vi "SI100_R1.vi"() -> ()   [LabVIEW 2022 SP3, in "SI100_ReactorTemperatureRise.lvclass"]
uses:
  SI100_ReactorTemperatureRise.lvclass
  SI100_ReactorTemperatureRise.lvclass/SI100_ReactorTemperatureRise.ctl
  SIClass/SIClass.lvclass
panel:
  out "SIClass out 4":refnum<class "SIClass.lvclass">
  out "SIClass out 3":refnum<class "SIClass.lvclass">
  out "SIClass out 2":refnum<class "SIClass.lvclass">
  out "SIClass out":refnum<class "SIClass.lvclass">
  in  "error in":errorcluster
  out "T-Rise 2nd Max":dbl
  in  "3 JEC20 CT951 XQ01":dbl
  in  "Loop ID 4":enum16{"10", "20", "30", "40"}(ring)
  in  "3 JEC20 CT954 XQ01":dbl
  in  "Loop ID 3":enum16{"10", "20", "30", "40"}(ring)
  in  "3 JEC20 CT953 XQ01":dbl
  in  "Loop ID 2":enum16{"10", "20", "30", "40"}(ring)
  in  "3 JEC10 CT952 XQ01":dbl
  in  "Loop ID":enum16{"10", "20", "30", "40"}(ring)
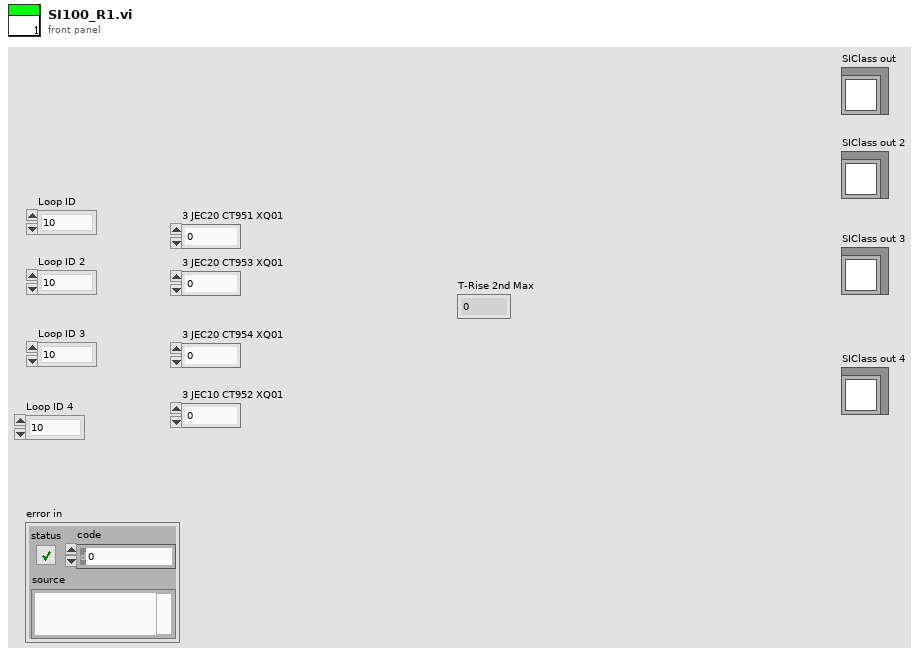
[diagram p1: front panel]
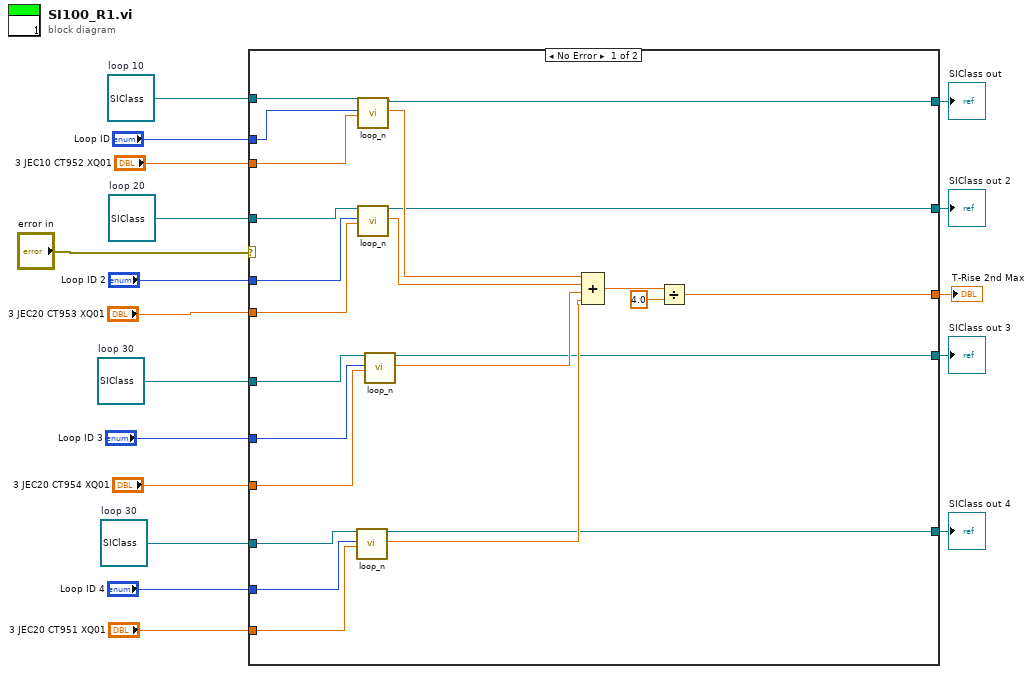
[diagram p0: block diagram]
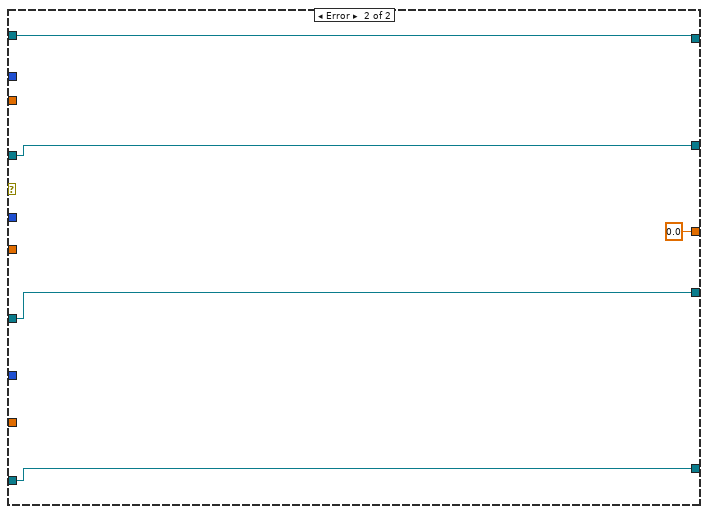
[diagram p2: hidden frame]
diagram:
  w7 = refnum<class "SIClass.lvclass"> refnum  # loop 30
  w10 = refnum<class "SIClass.lvclass"> refnum  # loop 30
  w15 = refnum<class "SIClass.lvclass"> refnum  # loop 20
  w18 = refnum<class "SIClass.lvclass"> refnum  # loop 10
  n1 = case shown="No Error" "error in" {
    tunnel: w18 -> [w41 w45]
    tunnel: "Loop ID" -> [w40 _]
    tunnel: "3 JEC10 CT952 XQ01" -> [w39 _]
    tunnel: w15 -> [w38 w44]
    tunnel: "Loop ID 2" -> [w37 _]
    tunnel: "3 JEC20 CT953 XQ01" -> [w36 _]
    tunnel: "3 JEC20 CT954 XQ01" -> [w35 _]
    tunnel: "Loop ID 3" -> [w34 _]
    tunnel: w10 -> [w33 w43]
    tunnel: "3 JEC20 CT951 XQ01" -> [w32 _]
    tunnel: "Loop ID 4" -> [w31 _]
    tunnel: w7 -> [w30 w42]
    tunnel: [w23 0.0] -> w6
    tunnel: [w22 w45] -> w4
    tunnel: [w21 w44] -> w3
    tunnel: [w20 w43] -> w2
    tunnel: [w19 w42] -> w1
    frame No Error {
      n2 = call-dynamic "loop_n.vi"("SIClass in"=w30, "Loop ID"=w31, "Input"=w32) -> ("SIClass out"=w19:refnum<class "SIClass.lvclass">, "Output"=w26:dbl)  [unwired: 14 in, 1 out]
      n3 = call-dynamic "loop_n.vi"("SIClass in"=w41, "Loop ID"=w40, "Input"=w39) -> ("SIClass out"=w22:refnum<class "SIClass.lvclass">, "Output"=w29:dbl)  [unwired: 14 in, 1 out]
      n4 = call-dynamic "loop_n.vi"("SIClass in"=w38, "Loop ID"=w37, "Input"=w36) -> ("SIClass out"=w21:refnum<class "SIClass.lvclass">, "Output"=w28:dbl)  [unwired: 14 in, 1 out]
      n5 = call-dynamic "loop_n.vi"("SIClass in"=w33, "Loop ID"=w34, "Input"=w35) -> ("SIClass out"=w20:refnum<class "SIClass.lvclass">, "Output"=w27:dbl)  [unwired: 14 in, 1 out]
      n6 = Compound Arithmetic op=ADD(w29, w28, w27, w26) -> (w25:dbl)
      n7 = Divide(x=w25, y=4.0) -> (x/y=w23:dbl)
    }
    frame Error {
    }
  }
  "T-Rise 2nd Max" <- w6
  "SIClass out" <- w4
  "SIClass out 2" <- w3
  "SIClass out 3" <- w2
  "SIClass out 4" <- w1
